vi "Do.vi"(8 "error in":errorcluster, 10 "Actor in":refnum<class "Actor.lvclass">, 11 "Request Data Msg":refnum<class "Request Data Msg.lvclass">) -> (0 "error out":errorcluster, 2 "Actor out":refnum<class "Actor.lvclass">)   [LabVIEW 2014, in "Request Data Msg.lvclass"]
doc: "(<B>Filename</B>: Actor Framework.lvlib:Message.lvclass:Do.vi)\n\nDefines what a message does when it is received by an actor. Generally, a message instructs an actor to invoke one of its methods.\n\nBy default, this method does nothing. A child class must override it to define behavior. Create a child class by using the Actor Framework Message Maker dialog box."
uses:
  Request Data Msg.lvclass
  <vilib>/ActorFramework/Actor/Actor.lvclass
  DAQ Device/DAQ Device.lvclass
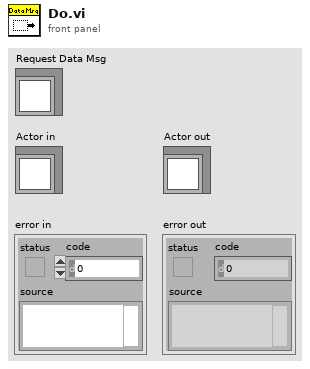
[diagram p1: front panel]
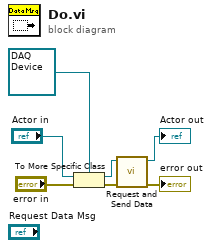
[diagram p0: block diagram]
diagram:
  n1 = To More Specific Class(target class=refnum<class "DAQ Device.lvclass"> refnum ("DAQ Device.lvlib:DAQ Device"), reference="Actor in", error in="error in") -> (specific class reference=w4:refnum<class "DAQ Device.lvclass">, error out=w3:errorcluster)
  n2 = call "Request and Send Data.vi"("error in"=w3, "DAQ Device in"=w4) -> ("error out"=→"error out":errorcluster, "DAQ Device out"=→"Actor out":refnum<class "DAQ Device.lvclass">)  [unwired: 8 in]
